vi "Update.vi"(6 "Table Name":string, 7 "condition":string, 8 "error in (no error)":errorcluster, 9 "Data List":string, 10 "ColumnName List":string, 11 "SQL Server in":refnum<class "SQL Server.lvclass">) -> (0 "error out":errorcluster, 2 "SQL Query":string, 3 "SQL Server out":refnum<class "SQL Server.lvclass">)   [LabVIEW 2021]
uses:
  SQL Server.lvclass
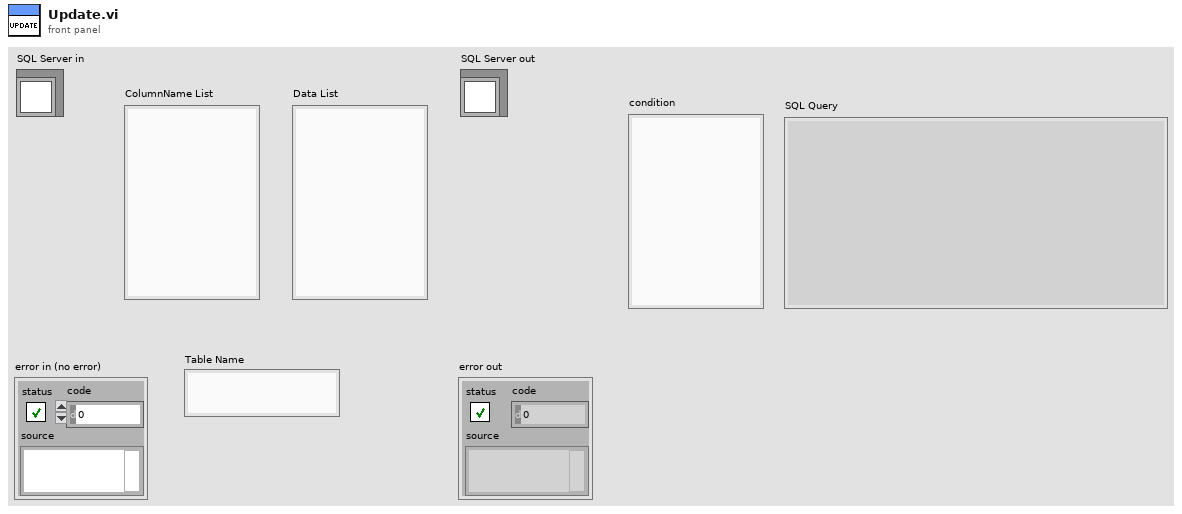
[diagram p1: front panel]
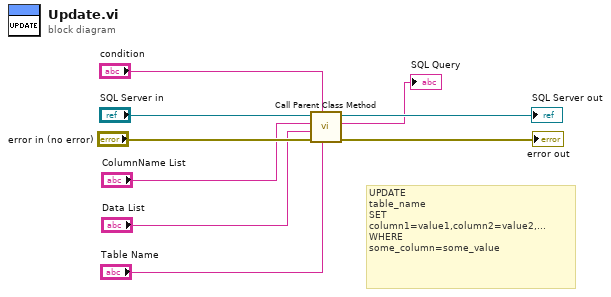
[diagram p0: block diagram]
diagram:
  # "UPDATE\ntable_name\nSET\ncolumn1=value1,column2=value2,...\nWHERE\nsome_column=some_value"
  n1 = call-parent "Call Parent Class Method"("Table Name"="Table Name", "condition"="condition", "error in (no error)"="error in (no error)", "Data List"="Data List", "ColumnName List"="ColumnName List", "DataBase_SQL in"="SQL Server in") -> ("error out"=→"error out":errorcluster, "SQL Query"=→"SQL Query":string, "DataBase_SQL out"=→"SQL Server out":refnum<class "SQL Server.lvclass">)  [unwired: 3 in]
